vi "Compress Images.vi"(7 "Front Panel":T1, 11 "Frame Data":T2(array[cluster])) -> (2 "Uncompressed Images":T1[](array[typedef]))   [LabVIEW 2024, in "VI Info.lvlib"]
doc: "This vi takes an array of image datas, and converts each of them into a Base64 compression string. It then returns an array with information for each image, including the rectangle, compressed string, the relative time it will appear for in a SVG, and the indexes for both the frame's owner and children. An array of the uncompressed image datas are also returned."
uses:
  VI Info.lvlib
  <vilib>/picture/picture.llb/imagedata.ctl
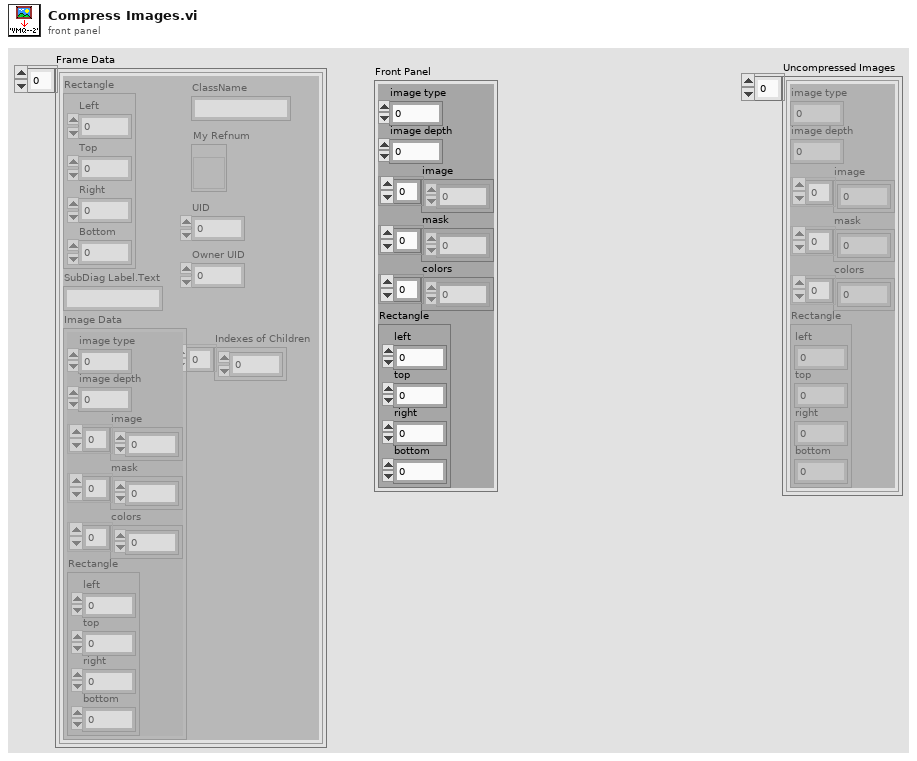
[diagram p1: front panel]
types:
  T1 = typedef "imagedata.ctl" = cluster{"image type":i32, "image depth":i32, "image":u8[], "mask":u8[], "colors":u32[], "Rectangle":cluster{"left":i16, "top":i16, "right":i16, "bottom":i16}}
  T2 = cluster{"Rectangle":cluster{"Left":i32, "Top":i32, "Right":u32, "Bottom":u32}, "SubDiag Label.Text":string, "Image Data":T1, "ClassName":string, "My Refnum":refnum<vi>, "UID":i32, "Owner UID":i32, "Indexes of Children":i32[]}[]
  T3 = cluster{"Rectangle":cluster{"Left":i32, "Top":i32, "Right":u32, "Bottom":u32}, "Image Data":T1, i32, "Indexes of Children":i32[]}
  T4 = cluster{"Width":i16, "Style":enum32{"Solid", "Dash", "Dot", "DashDot", "DashDotDot"}}
  T5 = cluster{"Left":i32, "Top":i32, "Right":u32, "Bottom":u32}
  T6 = cluster{"Rectangle":cluster{"Left":i32, "Top":i32, "Right":u32, "Bottom":u32}, "Image Data":T1, i32, i32[]}
  T7 = cluster{"left":i16, "top":i16, "right":i16, "bottom":i16}
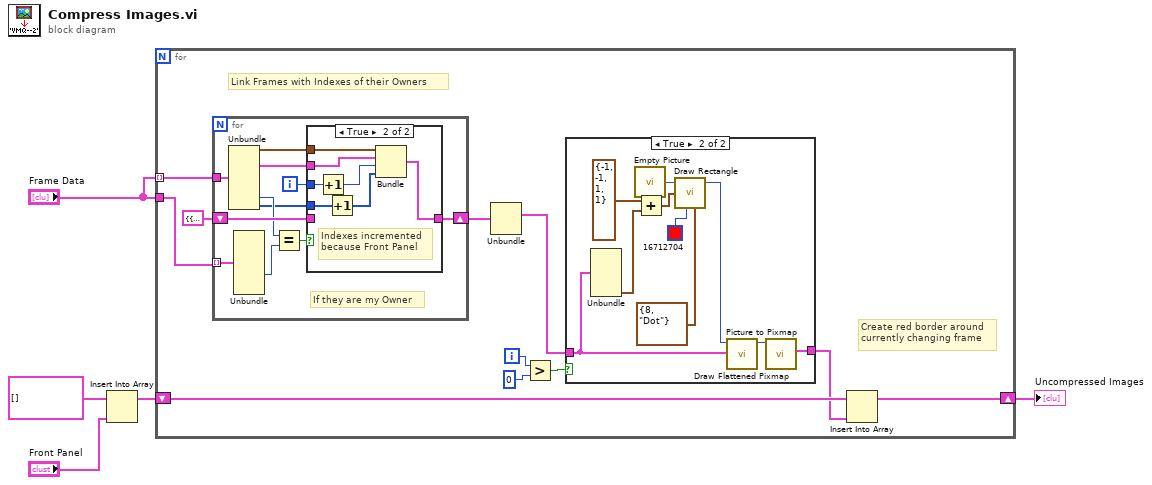
[diagram p0: block diagram]
diagram:
  n1 = Insert Into Array(array=T1[] [], new element="Front Panel") -> (w3:T1[])  [unwired: 1 in]
  n2 = for {
    tunnel: "Frame Data" -> [w15] mode=indexing
    tunnel: "Frame Data" -> [w14]
    shift-right: [w12] -> w2
    shift-left: w3 -> [w13]
    i -> [w9]
    # "Link Frames with Indexes of their Owners"
    # "Create red border around\ncurrently changing frame"
    n3 = for {
      tunnel: w14 -> [w26] mode=indexing
      tunnel: w15 -> [w27]
      shift-right: [w21] -> w16
      shift-left: T3 {"Rectangle"={"Left"=0, "Top"=0, "Right"=0, "Bottom"=0}, "Image Data"={"image type"=0, "image depth"=0, "image"=[], "mask"=[], "colors"=[], "Rectangle"={"left"=0, "top"=0, "right"=0, "bottom"=0}}, 0, "Indexes of Children"=[]} -> [w22]
      i -> [w18]
      # "If they are my Owner"
      n4 = Unbundle(w27) -> ("Rectangle"=w24:T5, "Image Data"=w23:T1, "Owner UID"=w20:i32, "Indexes of Children"=w17:i32[])  [unwired: 4 out]
      n5 = Unbundle(w26) -> ("UID"=w19:i32)  [unwired: 7 out]
      n6 = Equal?(x=w20, y=w19) -> (x = y?=w25:bool)
      n7 = case shown="True" w25 {
        tunnel: w24 -> [_ w35]
        tunnel: w23 -> [_ w34]
        tunnel: [w28 w33] -> w21
        tunnel: w22 -> [w28 _]
        tunnel: w18 -> [_ w32]
        tunnel: w17 -> [_ w30]
        frame False {
        }
        frame True {
          # "Indexes incremented\nbecause Front Panel"
          n8 = Increment(x=w32) -> (x+1=w31:i32)
          n9 = Increment(x=w30) -> (x+1=w29:i32[])
          n10 = Bundle("Rectangle"=w35, "Image Data"=w34, w31, w29) -> (w33:T6)  [unwired: 1 in]
        }
      }
    }
    n11 = Unbundle(w16) -> ("Image Data"=w11:T1)  [unwired: 3 out]
    n12 = Greater?(x=w9, y=0) -> (0:w10:bool)
    n13 = case shown="True" w10 {
      tunnel: w11 -> [w36 w39]
      tunnel: [w36 w37] -> w6
      frame False {
      }
      frame True {
        n14 = Unbundle(w39) -> ("Rectangle"=w45:T7)  [unwired: 5 out]
        n15 = call "Empty Picture"() -> ("empty picture"=w41:picture)
        n16 = Add(x=T5 {"Left"=-1, "Top"=-1, "Right"=1, "Bottom"=1}, y=w45) -> (x+y=w43:cluster{i32, i32, u32, u32})
        n17 = call <vilib>:"Draw Rectangle.vi"("picture"=w41, "rect"=w43, "color(black)"=u32 16712704, "pen"=T4 {"Width"=8, "Style"=enum."Dot"}) -> ("new picture"=w40:picture)  [unwired: 5 in]
        n18 = call <vilib>:"Draw Flattened Pixmap.vi"("image data"=w39, "picture"=w40) -> ("new picture"=w38:picture)  [unwired: 7 in]
        n19 = call <vilib>:"Picture to Pixmap.vi"("picture"=w38) -> ("image data"=w37:T1)  [unwired: 9 in, 1 out]
      }
    }
    n20 = Insert Into Array(array=w13, new element=w6) -> (w12:T1[])  [unwired: 1 in]
  }
  "Uncompressed Images" <- w2
